vi "set_Period_subvi.vi"(0 "Period":dbl, 1 "Combined Format? (False) in":bool, 5 "10-bit Addressing? (False) in":bool, 7 "No Stop? (False) in":bool, 9 "Aardvark Handle in":i32 min=0, 11 "error in (no error)":errorcluster, 12 "Address (0x50) in":u16=80 max=1023 format="%.0x") -> (3 "x 10ns 2":u8[](array[numeric]) format="%.0x", 4 "Boolean array 2":bool[](array[boolean]), 6 "dup Aardvark Handle 2":i32, 8 "Num Bytes Written 2":u16, 10 "Status 2":i32, 15 "error out":errorcluster)   [LabVIEW 2014]
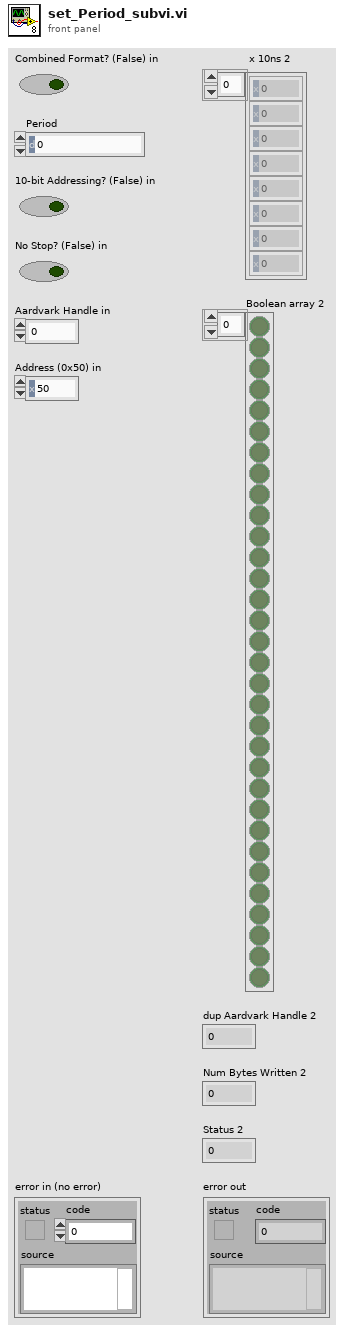
[diagram p1: front panel]
types:
  T1 = cluster{"unsigned byte array[0]":u8, "unsigned byte array[1]":u8, "unsigned byte array[2]":u8, "unsigned byte array[3]":u8, "unsigned byte array[4]":u8, "unsigned byte array[5]":u8, "unsigned byte array[6]":u8, "unsigned byte array[7]":u8, "unsigned byte array[8]":u8}
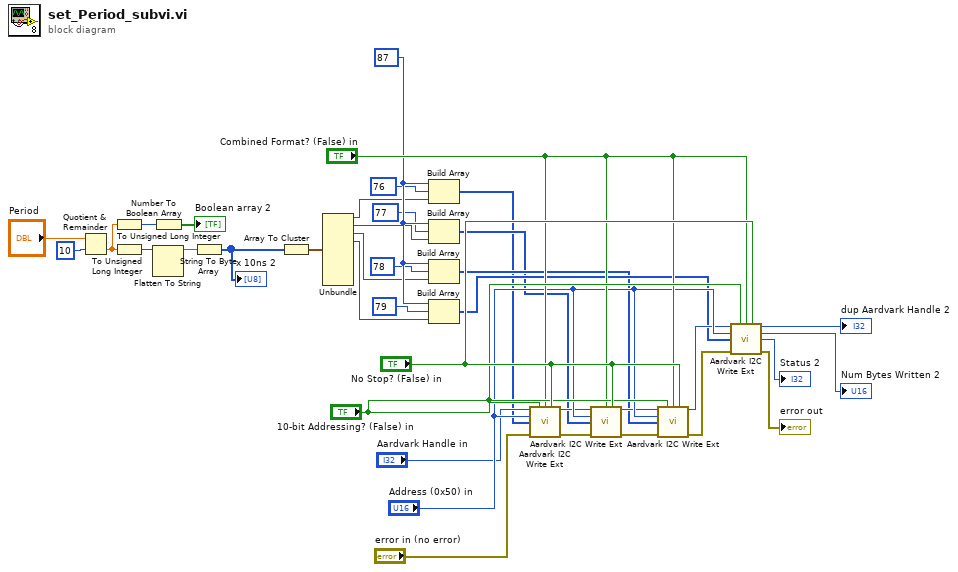
[diagram p0: block diagram]
diagram:
  w27 = u8 87
  n1 = Quotient & Remainder(x="Period", y=10) -> (floor(x/y)=w6:dbl)  [unwired: 1 out]
  n2 = To Unsigned Long Integer(number=w6) -> (unsigned 32bit integer=w3:u32)
  n3 = To Unsigned Long Integer(number=w6) -> (unsigned 32bit integer=w7:u32)
  n4 = Flatten To String(anything=w7) -> (data string=w5:string)  [unwired: 3 in, 2 out]
  n5 = Number To Boolean Array(number=w3) -> (Boolean array=→"Boolean array 2":bool[])
  n6 = String To Byte Array(string=w5) -> (unsigned byte array=w12:u8[])
  "x 10ns 2" <- w12
  n7 = Array To Cluster(array=w12) -> (cluster=w13:T1)
  n8 = Unbundle(w13) -> ("unsigned byte array[0]"=w15:u8, "unsigned byte array[1]"=w19:u8, "unsigned byte array[2]"=w20:u8, "unsigned byte array[3]"=w21:u8)  [unwired: 5 out]
  n9 = Build Array(w27, u16 76, w15) -> (w22:u16[])
  n10 = Build Array(w27, u16 77, w19) -> (w23:u16[])
  n11 = Build Array(w27, u16 78, w20) -> (w24:u16[])
  n12 = Build Array(w27, u16 79, w21) -> (w25:u16[])
  n13 = call <instrlib>:"Aardvark I2C Write Ext.vi"("Aardvark Handle"="Aardvark Handle in", "10-bit Addressing? (False)"="10-bit Addressing? (False) in", "Combined Format? (False)"="Combined Format? (False) in", "No Stop? (False)"="No Stop? (False) in", "Address (0x50)"="Address (0x50) in", "Data to Write"=w22, "error in (no error)"="error in (no error)") -> ("dup Aardvark Handle"=w29:i32, "error out"=w9:errorcluster)  [unwired: 5 in, 2 out]
  n14 = call <instrlib>:"Aardvark I2C Write Ext.vi"("Aardvark Handle"=w29, "Combined Format? (False)"="Combined Format? (False) in", "No Stop? (False)"="No Stop? (False) in", "Address (0x50)"="Address (0x50) in", "Data to Write"=w23, "error in (no error)"=w9) -> ("dup Aardvark Handle"=w30:i32, "error out"=w10:errorcluster)  [unwired: 6 in, 2 out]
  n15 = call <instrlib>:"Aardvark I2C Write Ext.vi"("Aardvark Handle"=w30, "10-bit Addressing? (False)"="10-bit Addressing? (False) in", "Combined Format? (False)"="Combined Format? (False) in", "No Stop? (False)"="No Stop? (False) in", "Address (0x50)"="Address (0x50) in", "Data to Write"=w24, "error in (no error)"=w10) -> ("dup Aardvark Handle"=w31:i32, "error out"=w11:errorcluster)  [unwired: 5 in, 2 out]
  n16 = call <instrlib>:"Aardvark I2C Write Ext.vi"("Aardvark Handle"=w31, "10-bit Addressing? (False)"="10-bit Addressing? (False) in", "Combined Format? (False)"="Combined Format? (False) in", "No Stop? (False)"="No Stop? (False) in", "Address (0x50)"="Address (0x50) in", "Data to Write"=w25, "error in (no error)"=w11) -> ("dup Aardvark Handle"=→"dup Aardvark Handle 2":i32, "Num Bytes Written"=→"Num Bytes Written 2":u16, "Status"=→"Status 2":i32, "error out"=→"error out":errorcluster)  [unwired: 5 in]
